vi "FC_Teams_at_Comp.vi"(8 "error constant":errorcluster, 10 "Event ID":string) -> (0 "error out":errorcluster, 2 "Array of Team Numbers":string[](array[string])=["118", "148", "231", "245", "457", "488", "499", "653", "704", "922", "1477", "1817", "2080", "2158", "2283", "2461", "2468", "2583", "2721", "2745", "2787", "2789", "2833", "2848", "2936", "2952", "2966", "2969", "2982", "2985", "3028", "2009", "3029", "3035", "3080", "3103", "3240", "3325", "3335", "3345", "3353", "3366", "3370", "3417", "3478", "3481", "3497", "3545", "3552", "3561", "3582", "3614", "3696", "3700", "3743", "3834", "3943", "3999", "4000", "4063", "4162", "4219", "4282", "4332"])   [LabVIEW 2013, in "FC_FIRST Client.lvlib"]
doc: "Given a competition ID#, this VI returns an array of the teams that will be present at that competition"
uses:
  FC_FIRST Client.lvlib
  <vilib>/regexp/Match Regular Expression.xnode
  <vilib>/httpClient/LabVIEWHTTPClient.lvlib
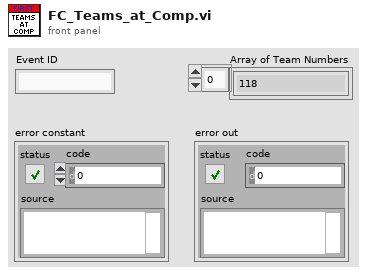
[diagram p1: front panel]
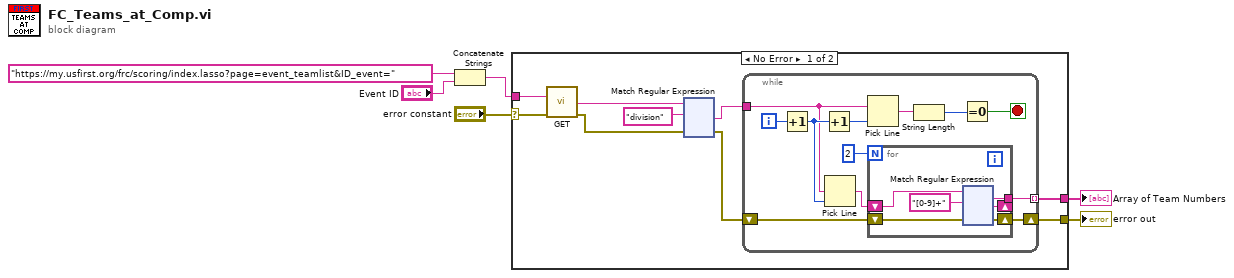
[diagram p0: block diagram]
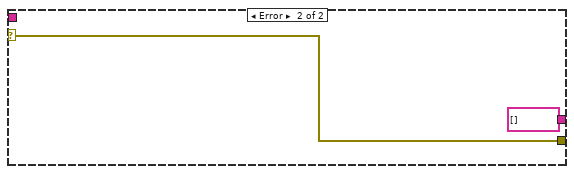
[diagram p2: hidden frame]
diagram:
  n1 = Concatenate Strings("https://my.usfirst.org/frc/scoring/index.lasso?page=event_teamlist&ID_event=" ("URL to List of Teams at Competition Base Path"), "Event ID") -> (w3:string)
  n2 = case shown="No Error" "error constant" {
    selector: "error constant" -> [w15 w256]
    tunnel: [w9 string[] []] -> w1
    tunnel: [w7 w256] -> w2
    tunnel: w3 -> [w14 _]
    frame No Error {
      n3 = call <vilib>:"GET.vi"("url"=w14, "error in (no error)"=w15) -> ("body"=w12:string, "error out"=w11:errorcluster)  [unwired: 10 in, 2 out]
      n4 = xnode "Match Regular Expression"("input string"=w12, "regular expression"="division", "error in"=w11) -> ("after match"=w10:string, "error out"=w8:errorcluster)  [unwired: 3 in, 3 out]
      n5 = while {
        tunnel: w10 -> [w135]
        tunnel: [w130] -> w9 mode=indexing
        shift-right: [w128] -> w7
        shift-left: w8 -> [w129]
        i -> [w138]
        stop <- w132 stop-if-true
        n6 = Increment(x=w138) -> (x+1=w136:i32)
        n7 = Increment(x=w136) -> (x+1=w137:i32)
        n8 = Pick Line(multi-line string=w135, line index=w136) -> (output string=w127:string)  [unwired: 1 in]
        n9 = Pick Line(multi-line string=w135, line index=w137) -> (output string=w134:string)  [unwired: 1 in]
        n10 = for {
          N: 2 -> [_]
          tunnel: [w143] -> w130
          shift-right: [w141] -> w128
          shift-left: w129 -> [w142]
          shift-right: [w140] -> _
          shift-left: w127 -> [w139]
          n11 = xnode "Match Regular Expression"("input string"=w139, "regular expression"="[0-9]+", "error in"=w142) -> ("whole match"=w143:string, "after match"=w140:string, "error out"=w141:errorcluster)  [unwired: 3 in, 2 out]
        }
        n12 = String Length(string=w134) -> (length=w133:i32)
        n13 = Equal To 0?(x=w133) -> (x = 0?=w132:bool)
      }
    }
    frame Error {
    }
  }
  "Array of Team Numbers" <- w1
  "error out" <- w2
